vi "Lower.vi"(8 "error in (no error)":errorcluster, 10 "Speed":dbl=-0.75 format="%#_13g", 11 "Gantry in":refnum<class "A3200.lvclass">) -> (0 "error out":errorcluster, 3 "Gantry out":refnum<class "A3200.lvclass">)   [LabVIEW 2016, in "A3200.lvclass"]
uses:
  A3200.lvclass
  Drivers/Aerotech A3200/Aerotech VIs.lvlib
  Drivers/Aerotech A3200/Motion/FreerunSingle.vi
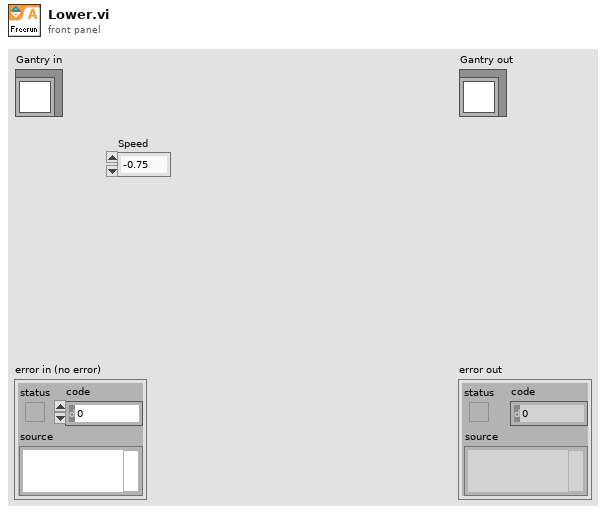
[diagram p1: front panel]
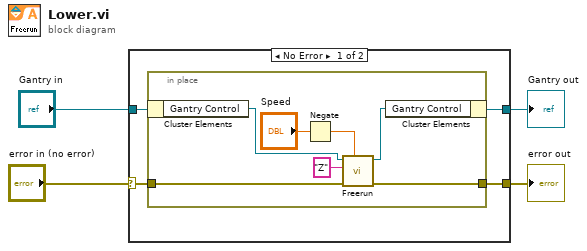
[diagram p0: block diagram]
diagram:
  n1 = case shown="No Error" "error in (no error)" {
    selector: "error in (no error)" -> [w6 w17]
    tunnel: "Gantry in" -> [w8 w16]
    tunnel: [w7 w16] -> w3
    tunnel: [w5 w17] -> w1
    frame No Error {
      n2 = in-place {
        in-place-border: w6 -> [w12]
        in-place-border: [w11] -> w5
        n3 = in-place-cluster #1(w8) -> ("Gantry Control"=w14:refnum<k24>)
        n4 = Negate(x="Speed") -> (-x=w9:dbl)
        n5 = call-poly "Freerun.vi"("speed"=w9, "error in (no error)"=w12, "axis name"="Z", "controller in"=w14) -> ("error out"=w11:errorcluster, "controller out"=w13:refnum<k24>)  [unwired: 6 in]
        n6 = in-place-cluster #1("Gantry Control"=w13) -> (w7:refnum<class "A3200.lvclass">)
      }
    }
    frame Error {
    }
  }
  "error out" <- w1
  "Gantry out" <- w3
